vi "DFD Probe Check MRate Filter.vi"(1 "multirate filter":T2={"mMRate_Structure"=enum."CIC", "mMRate_Mode"=0, "mMRate_Factor"=0, "mMRate_FIRParams"={"mMRate_FIR_H"=[], "mMRate_FIR_IsNyquist?"=FALSE, "mMRate_FIR_IsSymmetric?"=FALSE}, "mMRate_CICParams"={"mMRate_CIC_#Stage"=0, "mMRate_CIC_Lag"=0, "mMRate_CIC_Type"=enum."Lowpass"}, "mMRate_Order"=0, "mMRate_Version"="", "mMRate_Comments"="", "mMRate_RationalFactor"={"mMRate_L"=-1, "mMRate_M"=-1}, "mMRate_Fs"=1.0, "mMRate_Quantized?"=FALSE, "mMRate_QFilterGain"=1.0, "mMRate_CoefWl"=16, "mMRate_Scaling"={"mMRate_ScaleByPowerOf2?"=FALSE, "mMRate_ScaleType"=enum."Time Domain 1-Norm"}, "mMRate_InputWl"=0, "mMRate_OutputWl"=0, "mMRate_OutputMode"=enum."Nearest", "mMRate_MultMode"=enum."Truncated", "mMRate_BitPruning"=FALSE, "mMRate_GainWl"=16, "mMRate_OutputFwl"=0, "mMRate_SumIwl"=0, "mMRate_InputIwl "=16, "mMRate_SumWl"=32, "mMRate_CoefIwl"=0} {"mMRate_SumWl" min=1 max=32 step=1; "mMRate_InputIwl" min=1 max=32 step=1; "mMRate_GainWl" min=1 max=32 step=1; "mMRate_OutputWl" min=1 max=32 step=1; "mMRate_InputWl" min=1 max=32 step=1; "mMRate_CoefWl" min=1 max=32 step=1; "mMRate_Mode" items=["Default"=-1, "No Rate Change"=0, "Interpolation"=1, "Decimation"=2, "Interpolated"=3, "Rational"=4]}) -> (0 "Boolean":bool)   [LabVIEW 2017, in "NI_DigFilterLicensed.lvlib"]
uses:
  <vilib>/addons/Digital Filter Design/NI_DigFilterLicensed.lvlib
  <vilib>/addons/Digital Filter Design/_Objects.llb/DFD Multirate Filter Obj.ctl
  <vilib>/addons/Digital Filter Design/_Objects.llb/DFD Multirate Mode.ctl
  <vilib>/addons/Digital Filter Design/_Objects.llb/DFD Coef Norm Type.ctl
  <vilib>/addons/Digital Filter Design/_Objects.llb/DFD Round-off Mode.ctl
  <vilib>/addons/Digital Filter Design/_Objects.llb/DFD FXP MRate Multiply Mode.ctl
panel:
  in  "Tab Control":T1(tab)
  in  "filter gain":dbl format="%#_8g"
  out "quantized?":bool
  out "Mode":u16(ring) items=["No Rate Change", "Interpolation", "Decimation", "Interpolated", "Rational Resampling"]
  in  "M":i32=1
  in  "L":i32=1
  out "Structure":u16(ring)=2 items=["CIC", "FIR", "Invalid"]
  in  "Magnitude in dB":bool=TRUE
  out "Freq Resp":cluster{"f0":dbl, "df":dbl, "values":dbl[]}[](graph)
  in  "order":i32=-1
  out "coef":dbl[](graph)
  out "Type":u16(ring) items=["Lowpass", "Highpass"]
  in  "Lag":i32=-1
  in  "#Stage":i32=-1
  # "Quantized?"
  # "Filter Gain"
  # "Order"
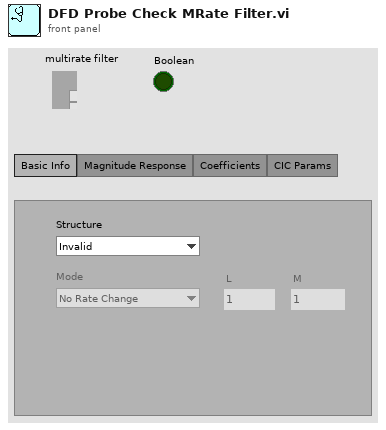
[diagram p1: front panel]
types:
  T1 = enum32{"Basic Info", "Magnitude Response", "Coefficients", "CIC Params"}
  T2 = typedef "NI_DigFilterLicensed.lvlib/DFD Multirate Filter Obj.ctl" = cluster{"mMRate_Structure":enum16{"CIC", "FIR", "IIR", "Lattice"}, "mMRate_Mode":T3, "mMRate_Factor":i32, "mMRate_FIRParams":cluster{"mMRate_FIR_H":dbl[], "mMRate_FIR_IsNyquist?":bool, "mMRate_FIR_IsSymmetric?":bool}, "mMRate_CICParams":cluster{"mMRate_CIC_#Stage":i32, "mMRate_CIC_Lag":i32, "mMRate_CIC_Type":enum16{"Lowpass", "Highpass"}}, "mMRate_Order":i32, "mMRate_Version":string, "mMRate_Comments":string, "mMRate_RationalFactor":cluster{"mMRate_L":i32, "mMRate_M":i32}, "mMRate_Fs":dbl, "mMRate_Quantized?":bool, "mMRate_QFilterGain":dbl, "mMRate_CoefWl":i16, "mMRate_Scaling":cluster{"mMRate_ScaleByPowerOf2?":bool, "mMRate_ScaleType":T4}, "mMRate_InputWl":i16, "mMRate_OutputWl":i16, "mMRate_OutputMode":T5, "mMRate_MultMode":T6, "mMRate_BitPruning":bool, "mMRate_GainWl":i16, "mMRate_OutputFwl":i16, "mMRate_SumIwl":i16, "mMRate_InputIwl ":i16, "mMRate_SumWl":i16, "mMRate_CoefIwl":i16}
  T3 = typedef "NI_DigFilterLicensed.lvlib/DFD Multirate Mode.ctl" = i16
  T4 = typedef "NI_DigFilterLicensed.lvlib/DFD Coef Norm Type.ctl" = enum16{"No Norm", "Time Domain 1-Norm", "Time Domain 2-Norm", "Time Domain Inf-Norm"}
  T5 = typedef "NI_DigFilterLicensed.lvlib/DFD Round-off Mode.ctl" = enum16{"Nearest", "Truncation"}
  T6 = typedef "NI_DigFilterLicensed.lvlib/DFD FXP MRate Multiply Mode.ctl" = enum16{"Truncated", "Full"}
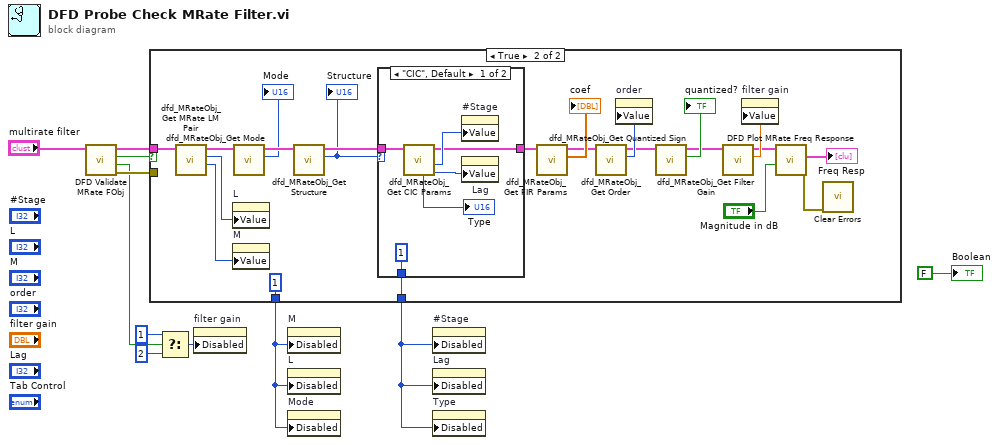
[diagram p0: block diagram]
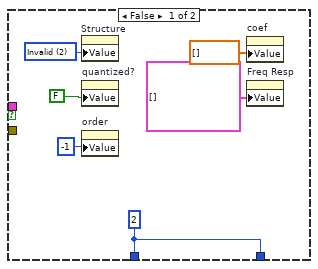
[diagram p2: hidden frame]
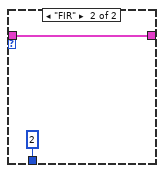
[diagram p3: hidden frame]
diagram:
  n1 = call <vilib>:"DFD Validate MRate FObj.vi"("multirate filter in"="multirate filter") -> ("error out"=w8:errorcluster, "is valid FXP?"=w6:bool, "is valid FLP?"=w9:bool, "multirate filter out"=w7:T2)  [unwired: 1 in, 6 out]
  n2 = case shown="True" w9 {
    tunnel: w8 -> [_ _]
    tunnel: w7 -> [_ w39]
    tunnel: [w14 w20] -> w2
    tunnel: [w14 u8 1 ("Disabled")] -> w1
    frame False {
      w14 = u8 2 ("Disabled")
      w17 = u16 2 items=["CIC", "FIR", "Invalid"] ("Structure")
      n3 = property on="Structure" class="Ring (strict)"("Value"=w17) -> ()  [unwired: 2 in, 2 out]
      n4 = property on="quantized?" class="Bool (strict)"("Value"=FALSE ("quantized?")) -> ()  [unwired: 2 in, 2 out]
      n5 = property on="order" class="DigNum (strict)"("Value"=-1 ("order")) -> ()  [unwired: 2 in, 2 out]
      n6 = property on="coef" class="WFGraph (strict)"("Value"=dbl[] [] ("coef")) -> ()  [unwired: 2 in, 2 out]
      n7 = property on="Freq Resp" class="WFGraph (strict)"("Value"=cluster{"f0":dbl, "df":dbl, "values":dbl[]}[] [] ("Freq Resp")) -> ()  [unwired: 2 in, 2 out]
    }
    frame True {
      n8 = call <vilib>:"dfd_MRateObj_Get MRate LM Pair.vi"("multirate filter in"=w39) -> ("M"=w37:i32, "L"=w38:i32, "dup multirate filter"=w36:T2)  [unwired: 1 in, 7 out]
      n9 = property on="L" class="DigNum (strict)"("Value"=w38) -> ()  [unwired: 2 in, 2 out]
      n10 = property on="M" class="DigNum (strict)"("Value"=w37) -> ()  [unwired: 2 in, 2 out]
      n11 = call <vilib>:"dfd_MRateObj_Get Mode.vi"("multirate filter in"=w36) -> ("mode"=→"Mode":T3, "dup multirate filter"=w35:T2)  [unwired: 9 out]
      n12 = call <vilib>:"dfd_MRateObj_Get Structure.vi"("multirate filter in"=w35) -> ("structure"=w33:enum16{"CIC", "FIR", "IIR", "Lattice"}, "dup multirate filter"=w34:T2)  [unwired: 9 out]
      "Structure" <- w33
      n13 = case shown="\"CIC\", Default" w33 {
        tunnel: w34 -> [w45 w47]
        tunnel: [w41 w47] -> w32
        tunnel: [u8 1 ("Disabled") u8 2 ("Disabled")] -> w20
        frame "CIC", Default {
          n14 = call <vilib>:"dfd_MRateObj_Get CIC Params.vi"("multirate filter in"=w45) -> ("lag"=w43:i32, "# stages"=w44:i32, "dup multirate filter"=w41:T2, "type"=→"Type":enum16{"Lowpass", "Highpass"})  [unwired: 7 out]
          n15 = property on="#Stage" class="DigNum (strict)"("Value"=w44) -> ()  [unwired: 2 in, 2 out]
          n16 = property on="Lag" class="DigNum (strict)"("Value"=w43) -> ()  [unwired: 2 in, 2 out]
        }
        frame "FIR" {
        }
      }
      n17 = call <vilib>:"dfd_MRateObj_Get FIR Params.vi"("multirate filter in"=w32) -> ("h(n)"=→"coef":dbl[], "dup multirate filter"=w30:T2)  [unwired: 9 out]
      n18 = call <vilib>:"dfd_MRateObj_Get Order.vi"("multirate filter in"=w30) -> ("order"=w29:i32, "dup multirate filter"=w28:T2)  [unwired: 9 out]
      n19 = property on="order" class="DigNum (strict)"("Value"=w29) -> ()  [unwired: 2 in, 2 out]
      n20 = call <vilib>:"dfd_MRateObj_Get Quantized Sign.vi"("multirate filter in"=w28) -> ("is Quantized?"=→"quantized?":bool, "dup multirate filter"=w26:T2)  [unwired: 9 out]
      n21 = call <vilib>:"dfd_MRateObj_Get Filter Gain.vi"("multirate filter in"=w26) -> ("gain"=w25:dbl, "dup multirate filter"=w24:T2)  [unwired: 9 out]
      n22 = property on="filter gain" class="DigNum (strict)"("Value"=w25) -> ()  [unwired: 2 in, 2 out]
      n23 = call <vilib>:"DFD Plot MRate Freq Response.vi"("dB on? (T)"="Magnitude in dB", "multirate filter in"=w24) -> ("error out"=w22:errorcluster, "magnitude response"=→"Freq Resp":cluster{"f0":dbl, "df":dbl, "values":dbl[]}[])  [unwired: 5 in, 3 out]
      n24 = call <vilib>:"Clear Errors.vi"("error in (no error)"=w22) -> ()  [unwired: 1 in, 6 out]
    }
  }
  n25 = Select(t=u8 1 ("Disabled"), s=w6, f=u8 2 ("Disabled")) -> (s? t:f=w5:u8)
  n26 = property on="filter gain" class="DigNum (strict)"("Disabled"=w5) -> ()  [unwired: 2 in, 2 out]
  n27 = property on="M" class="DigNum (strict)"("Disabled"=w1) -> ()  [unwired: 2 in, 2 out]
  n28 = property on="L" class="DigNum (strict)"("Disabled"=w1) -> ()  [unwired: 2 in, 2 out]
  n29 = property on="Mode" class="Ring (strict)"("Disabled"=w1) -> ()  [unwired: 2 in, 2 out]
  n30 = property on="#Stage" class="DigNum (strict)"("Disabled"=w2) -> ()  [unwired: 2 in, 2 out]
  n31 = property on="Lag" class="DigNum (strict)"("Disabled"=w2) -> ()  [unwired: 2 in, 2 out]
  n32 = property on="Type" class="Ring (strict)"("Disabled"=w2) -> ()  [unwired: 2 in, 2 out]
  "Boolean" <- FALSE ("Boolean")
